vi "Blocking Performance Test Managment.vi"() -> ()   [LabVIEW 2013]
doc: "This VI will run the blobking performance tests at all required blocking frequency. See the below pseudo code for a description of its operation.\n\n1. Two test signals are fed to the EUT (equipment under test) input port: \na. Wanted signal: \ni. Modulated carrier, packets transmitted at the mid operating frequency = 2426 \nMHz, with 37-octets PRBS9 (pseudo random bit sequence 9) payload. Signal \nlevel of the wanted signal at the EUT input port shall be as defined below. \nb. Blocking signal: \ni. Sinusoidal, un-modulated carrier transmitted at a blocker frequency of fblocker \n= 30MHz. Signal level of the blocker signal at the EUT input port shall be as \ndefined in Table 1. \n2. If the PER (packet error rate) exceeds the minimum requirement, the frequency is recorded as \nfbf_1. \n3. Repeat steps for 1) and 2) for 30MHz = fblocker = 12.75GHz with the measurement \nfrequency resolution defined in Table 1. \n4. fblocker n+1 = fblocker_n + measurement frequency resolution (n=0,1,2…). \n5. The PER measurement is repeated for all recorded frequencies in 2) but with -50dBm blocker \nlevel at the EUT input ports. If the PER exceeds the minimum requirement, the frequency is \nrecorded as fbf_2. \nInterference signal frequency | Wanted signal level at EUT input port | Blocking signal level at EUT input port | Measurement frequency resolution \n30 – 2000 MHz | -67dBm | -30dBm | 10 MHz \n2003 – 2399 MHz | -67dBm | -35dBm | 3 MHz \n2484 – 2997 MHz | -67dBm | -35dBm | 3 MHz \n3000 MHz – 12.75 GHz | -67dBm | -30dBm | 25 MHz"
uses:
  Sub VIs/Master Test Parameters.ctl
  Sub VIs/Test Results Display Cluster.ctl
  Sub VIs/Pass Weighting.ctl
  Sub VIs/Test Managment Application Queue Control Cluster.ctl
  Sub VIs/Test Managment Application Queue Control.ctl
  Sub VIs/Results FGV Command.ctl
  Sub VIs/UUT Control Command.ctl
  Sub VIs/Test Parameters.ctl
  Sub VIs/Globals/Test Criteria Global.vi
panel:
  in  "Speed Throttle":bool
  out "Packets Sent":dbl format="%#.0f%%"
  in  "Result Emulation":T1=enum."Random"
  out "PER Pass Rate":dbl min=0.0 max=100.0 format="%#_g%%"
  out "Testing In Progress":bool
  out "State":string caption="Current Application State"
  out "Test Result":bool
  out "fbf_2 Pass Criteria":i32
  out "fbf_1 Pass Criteria":i32
  out "fbf_2":i32 caption="fbf_2 Results"
  out "fbf_1":i32 caption="fbf_1 Results"
  out "Array of Results":T2[](array[typedef]) {"Percentage Error Rates" format="%.1f%%"; "Test Frequency" format="%.0f MHz"}
  out "Freq. Under Test":u32 caption="Current frequency Under Test" format="%.0fMHz"
  out "Array of tests":T3[](array[typedef]) {"Measurement Res." format="%.0f MHz"; "Blocking Signal" format="%#_gdBm"; "Wanted Signal" format="%#_gdBm"; "Upper Frequency" format="%.0f MHz"; "Lower Frequency" format="%.0f MHz"}
  # "Blocking Performance Automated Test"
  # "Test Freq."
  # "Rcved Packets"
  # "Result"
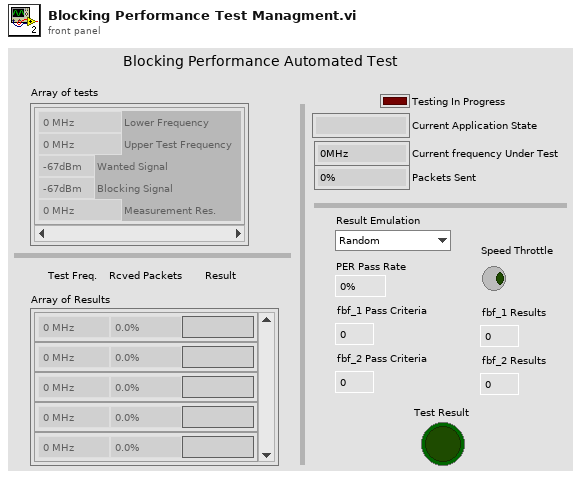
[diagram p1: front panel]
types:
  T1 = typedef "Pass Weighting.ctl" = enum16{"Always Pass", "Always Fail", "Always 30%", "Always 31%", "Random"}
  T2 = typedef "Test Results Display Cluster.ctl" = cluster{"Test Frequency":u32, "Percentage Error Rates":dbl, "Results":string}
  T3 = typedef "Master Test Parameters.ctl" = cluster{"Lower Frequency":u32, "Upper Frequency":u32, "Wanted Signal":dbl, "Blocking Signal":dbl, "Measurement Res.":u32}
  T4 = typedef "Test Managment Application Queue Control Cluster.ctl" = cluster{"State":T5, "Data":string}
  T5 = typedef "Test Managment Application Queue Control.ctl" = enum16{"Initialise", "Read Test Parameters", "Check for Correct UUT", "Round 1", "Set Blocking Signal Level", "Round 2", "Return Results", "Store Results", "End"}
  T6 = typedef "Results FGV Command.ctl" = enum16{"Add Result", "Return All", "Return fbf_1", "Return fbf_2", "Replace", "Clear All"}
  T7 = typedef "UUT Control Command.ctl" = enum16{"Initialise packet count", "Read Packet Count", "Return Temperature", "Return Operating Voltage"}
  T8 = typedef "Test Parameters.ctl" = cluster{"Interference sig. freq.":u32, "Wanted Signal":dbl, "Blocking Signal":dbl, "Measurement res.":u32}
  T9 = typedef "Test Results Cluster.ctl" = cluster{"Test Frequency":u32, "Received Packets":u32, "Results":string, "Test Paramaters":T8}
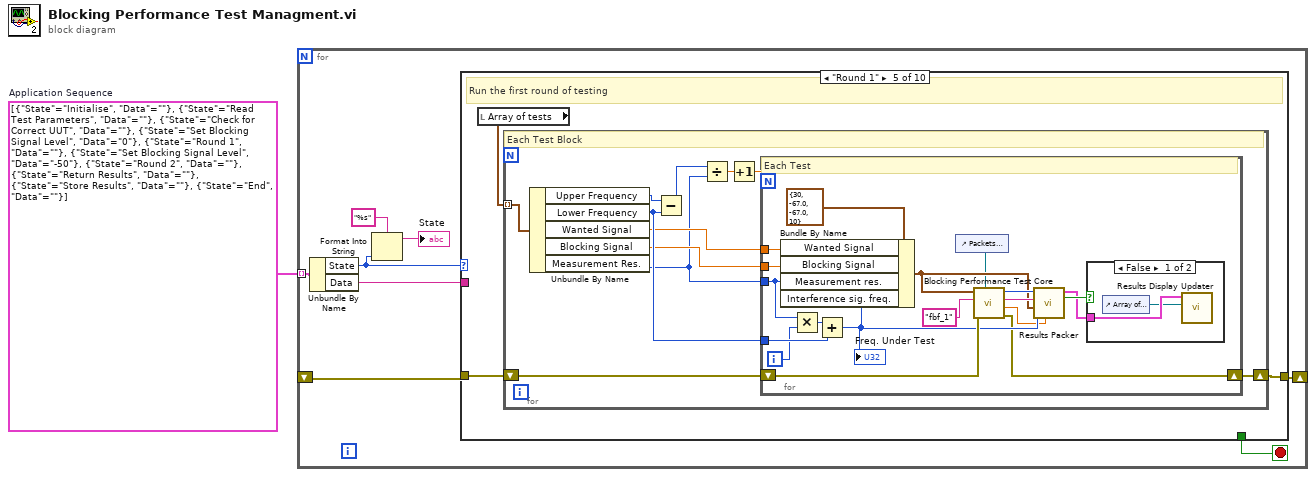
[diagram p0: block diagram]
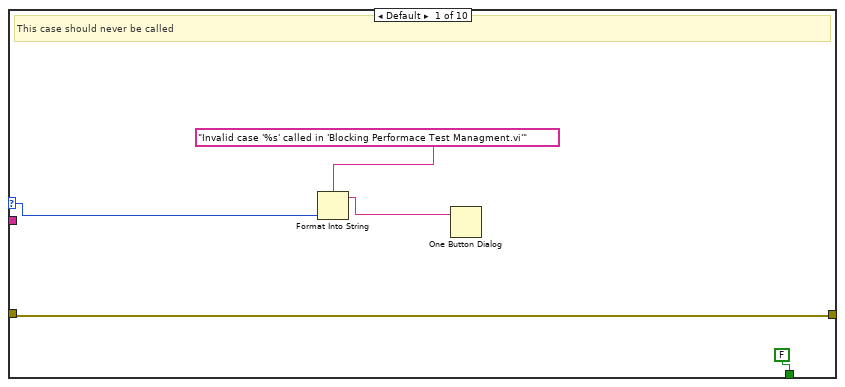
[diagram p2: hidden frame]
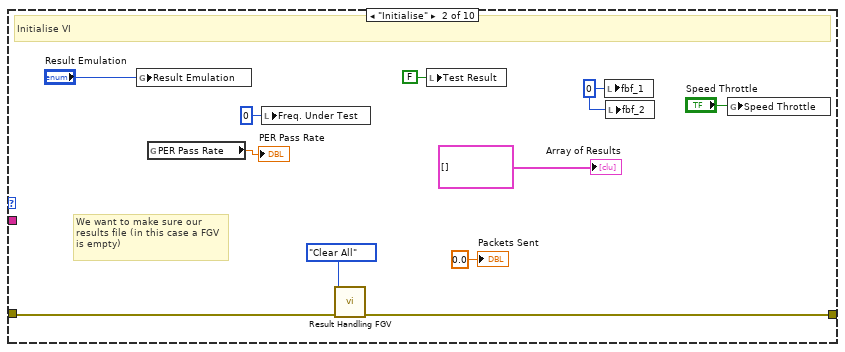
[diagram p3: hidden frame]
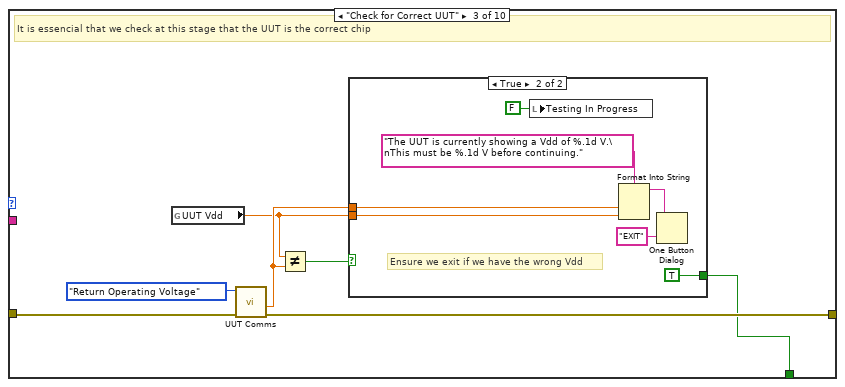
[diagram p4: hidden frame]
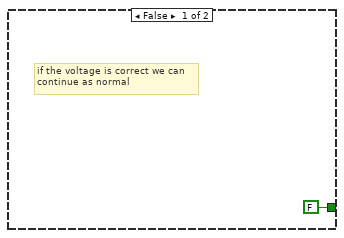
[diagram p5: hidden frame]
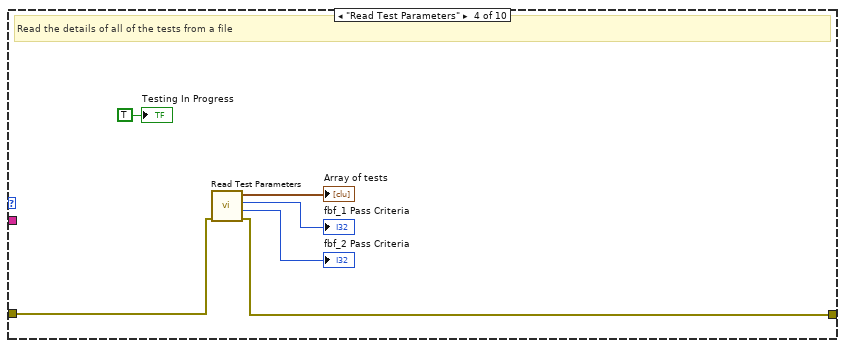
[diagram p6: hidden frame]
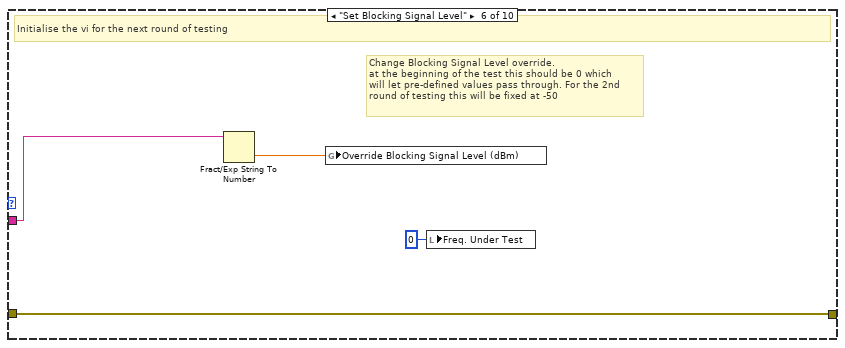
[diagram p8: hidden frame]
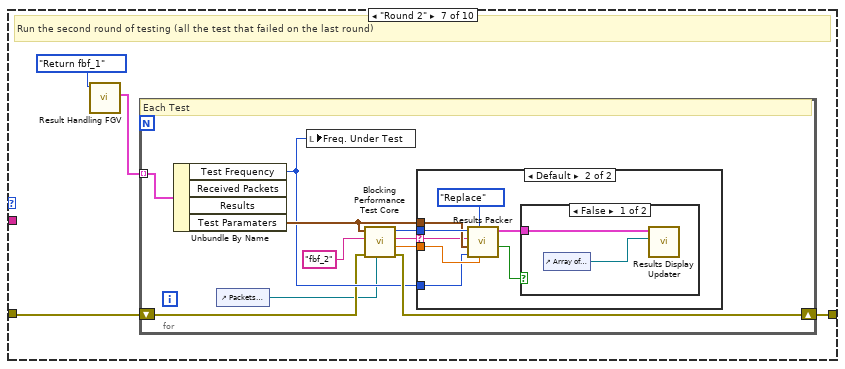
[diagram p9: hidden frame]
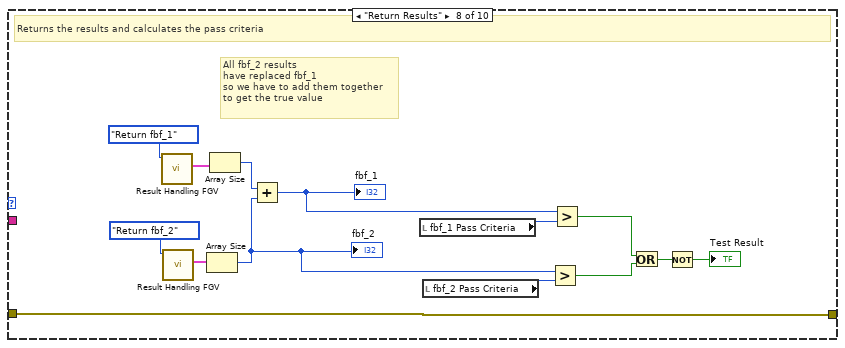
[diagram p12: hidden frame]
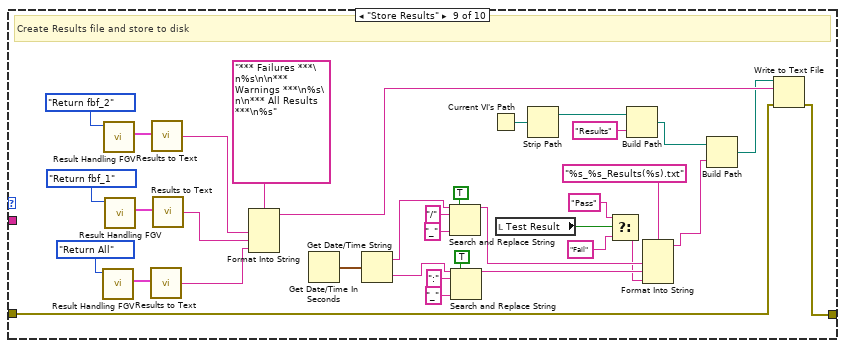
[diagram p13: hidden frame]
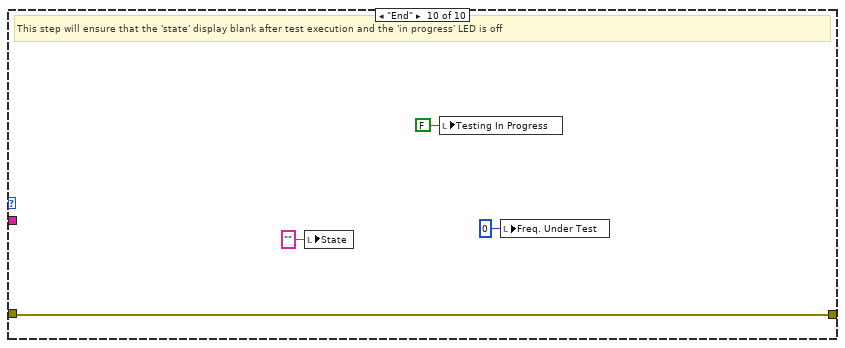
[diagram p14: hidden frame]
diagram:
  w1 = T4[] [{"State"=enum."Initialise", "Data"=""}, {"State"=enum."Read Test Parameters", "Data"=""}, {"State"=enum."Check for Correct UUT", "Data"=""}, {"State"=enum."Set Blocking Signal Level", "Data"="0"}, {"State"=enum."Round 1", "Data"=""}, {"State"=enum."Set Blocking Signal Level", "Data"="-50"}, {"State"=enum."Round 2", "Data"=""}, {"State"=enum."Return Results", "Data"=""}, {"State"=enum."Store Results", "Data"=""}, {"State"=enum."End", "Data"=""}]  # Application Sequence
  n1 = for {
    shift-right: [w9] -> _
    shift-left: _ -> [w8]
    tunnel: w1 -> [w6] mode=indexing
    stop <- w7 stop-if-true
    n2 = Unbundle By Name(w6) -> ("State"=w3:T5, "Data"=w4:string)
    n3 = Format Into String(format string="%s", w3) -> (resulting string=→"State":string)  [unwired: 2 in, 1 out]
    n4 = case shown="\"Round 1\"" w3 {
      selector: w3 -> [w11 _ _ _ _ _ _ _ _ _]
      tunnel: [w14 w23 w30 w44 w48 w83 w88 w111 w126 w161] -> w9
      tunnel: w8 -> [w14 w24 w31 w45 w47 w83 w87 w111 w127 w161]
      tunnel: [FALSE _ w28 _ _ _ _ _ _ _] -> w7
      tunnel: w4 -> [_ _ _ _ _ w82 _ _ _ _]
      frame Default {
        # "This case should never be called"
        n5 = Format Into String(format string="Invalid case '%s' called in 'Blocking Performace Test Managment.vi'" ("message"), w11) -> (resulting string=w12:string)  [unwired: 2 in, 1 out]
        n6 = One Button Dialog(message=w12) -> ()  [unwired: 1 in, 1 out]
      }
      frame "Initialise" {
        w21 = 0 ("fbf_1")
        # "We want to make sure our\nresults file (in this case a FGV\nis empty)"
        # "Initialise VI"
        n7 = global write "Test Criteria Global.vi" "Result Emulation"("Result Emulation") -> ()
        n8 = global read "Test Criteria Global.vi" "PER Pass Rate"() -> (→"PER Pass Rate":dbl)
        n9 = local write "Freq. Under Test"(u32 0 ("Freq. Under Test")) -> ()
        n10 = call "Result Handling FGV.vi"("error in"=w24, "Command"=Results_FGV_Command."Clear All") -> ("error out"=w23:errorcluster)  [unwired: 8 in, 1 out]
        n11 = local write "Test Result"(FALSE ("Test Result")) -> ()
        n12 = local write "fbf_1"(w21) -> ()
        n13 = local write "fbf_2"(w21) -> ()
        n14 = global write "Test Criteria Global.vi" "Speed Throttle"("Speed Throttle") -> ()
        "Packets Sent" <- 0.0 ("Packets Sent")
        "Array of Results" <- T2[] [] ("Results (Disp.)")
      }
      frame "Check for Correct UUT" {
        # "It is essencial that we check at this stage that the UUT is the correct chip"
        n15 = global read "Test Criteria Global.vi" "UUT Vdd"() -> (w26:dbl)
        n16 = call "UUT Comms.vi"("error in"=w31, "Command"=UUT_Control_Command."Return Operating Voltage") -> ("error out"=w30:errorcluster, "Vdd"=w27:dbl)  [unwired: 6 in, 2 out]
        n17 = Not Equal?(x=w26, y=w27) -> (x != y?=w29:bool)
        n18 = case shown="True" w29 {
          tunnel: [FALSE TRUE] -> w28
          tunnel: w27 -> [_ w36]
          tunnel: w26 -> [_ w35]
          frame False {
            # "if the voltage is correct we can\ncontinue as normal"
          }
          frame True {
            # "Ensure we exit if we have the wrong Vdd"
            n19 = local write "Testing In Progress"(FALSE ("Testing In Progress")) -> ()
            n20 = Format Into String(format string="The UUT is currently showing a Vdd of %.1d V.\nThis must be %.1d V before continuing.", w36, w35) -> (resulting string=w37:string)  [unwired: 2 in, 1 out]
            n21 = One Button Dialog(message=w37, button name ("OK")="EXIT") -> ()  [unwired: 1 out]
          }
        }
      }
      frame "Read Test Parameters" {
        # "Read the details of all of the tests from a file"
        n22 = call "Read Test Parameters.vi"("error in"=w45) -> ("error out"=w44:errorcluster, "fbf_2 Pass Criteria"=→"fbf_2 Pass Criteria":i32, "fbf_1 Pass Criteria"=→"fbf_1 Pass Criteria":i32, "Array of tests"=→"Array of tests":T3[])  [unwired: 7 in]
        "Testing In Progress" <- TRUE ("Testing In Progress")
      }
      frame "Round 1" {
        # "Run the first round of testing"
        n23 = local read "Array of tests"() -> (w49:T3[])
        n24 = for {
          tunnel: w49 -> [w60] mode=indexing
          shift-right: [w55] -> w48
          shift-left: w47 -> [w54]
          # "Each Test Block"
          n25 = Unbundle By Name(w60) -> ("Upper Frequency"=w59:u32, "Lower Frequency"=w58:u32, "Wanted Signal"=w57:dbl, "Blocking Signal"=w56:dbl, "Measurement Res."=w52:u32)
          n26 = Subtract(x=w59, y=w58) -> (x-y=w53:u32)
          n27 = Divide(x=w53, y=w52) -> (x/y=w51:dbl)
          n28 = Increment(x=w51) -> (x+1=w50:dbl)
          n29 = for {
            N: w50 -> [_]
            tunnel: w58 -> [w78]
            tunnel: w57 -> [w77]
            tunnel: w56 -> [w76]
            tunnel: w52 -> [w74]
            shift-right: [w65] -> w55
            shift-left: w54 -> [w75]
            i -> [w73]
            # "Each Test"
            n30 = Multiply(x=w74, y=w73) -> (x*y=w72:u32)
            n31 = Add(x=w72, y=w78) -> (x+y=w68:u32)
            "Freq. Under Test" <- w68
            n32 = Bundle By Name(cluster=T8 {"Interference sig. freq."=30, "Wanted Signal"=-67.0, "Blocking Signal"=-67.0, "Measurement res."=10} ("Test Paramaters"), "Wanted Signal"=w77, "Blocking Signal"=w76, "Measurement res."=w74, "Interference sig. freq."=w68) -> (w67:T8)
            n33 = control-ref of="Packets Sent"() -> (w62:refnum<vi>)
            n34 = call "Blocking Performance Test Core.vi"("Packets Sent"=w62, "error in"=w75, "test run"="fbf_1", "Test Paramaters"=w67) -> ("error out"=w65:errorcluster, "PER"=w66:dbl, "Results"=w71:string, "received Packets"=w70:u32)  [unwired: 4 in]
            n35 = call "Results Packer.vi"("PER"=w66, "Test Frequency"=w68, "Test Paramaters"=w67, "Results"=w71, "received Packets"=w70) -> ("Pass"=w64:bool, "Test Result Display Cluster"=w61:T2)  [unwired: 4 in, 1 out]
            n36 = case shown="False" w64 {
              tunnel: w61 -> [w80 _]
              frame False {
                n37 = control-ref of="Array of Results"() -> (w79:refnum<vi>)
                n38 = call "Results Display Updater.vi"("Array of Results Reference"=w79, "New Results"=w80) -> ()  [unwired: 10 in]
              }
              frame True {
              }
            }
          }
        }
      }
      frame "Set Blocking Signal Level" {
        # "Change Blocking Signal Level override.\nat the beginning of the test this should be 0 which\nwill let pre-defined values pass through. For the 2nd\nround of testing this will be fixed at -50"
        # "Initialise the vi for the next round of testing"
        n39 = Fract/Exp String To Number(string=w82) -> (number=w81:dbl)  [unwired: 3 in, 1 out]
        n40 = global write "Test Criteria Global.vi" "Override Blocking Signal Level (dBm)"(w81) -> ()
        n41 = local write "Freq. Under Test"(u32 0 ("Freq. Under Test")) -> ()
      }
      frame "Round 2" {
        # "Run the second round of testing (all the test that failed on the last round)"
        n42 = call "Result Handling FGV.vi"("Command"=Results_FGV_Command."Return fbf_1") -> ("Result Array"=w85:T9[])  [unwired: 9 in, 1 out]
        n43 = for {
          shift-right: [w96] -> w88
          shift-left: w87 -> [w90]
          tunnel: w85 -> [w95] mode=indexing
          # "Each Test"
          n44 = Unbundle By Name(w95) -> ("Test Frequency"=w92:u32, "Test Paramaters"=w94:T8)  [unwired: 2 out]
          n45 = control-ref of="Packets Sent"() -> (w89:refnum<vi>)
          n46 = local write "Freq. Under Test"(w92) -> ()
          n47 = call "Blocking Performance Test Core.vi"("Packets Sent"=w89, "error in"=w90, "test run"="fbf_2", "Test Paramaters"=w94) -> ("error out"=w96:errorcluster, "PER"=w97:dbl, "Results"=w91:string, "received Packets"=w98:u32)  [unwired: 4 in]
          n48 = case shown="Default" w91 {
            selector: w91 -> [_ w101]
            tunnel: w98 -> [_ w106]
            tunnel: w97 -> [_ w105]
            tunnel: w94 -> [_ w104]
            tunnel: w92 -> [_ w103]
            frame "Pass" {
              # "If the test now\npasses we leave\nthe results alone"
            }
            frame Default {
              n49 = call "Results Packer.vi"("PER"=w105, "Command (Add)"=Results_FGV_Command."Replace" ("Command"), "Test Frequency"=w103, "Test Paramaters"=w104, "Results"=w101, "received Packets"=w106) -> ("Pass"=w100:bool, "Test Result Display Cluster"=w99:T2)  [unwired: 3 in, 1 out]
              n50 = case shown="False" w100 {
                tunnel: w99 -> [w108 _]
                frame False {
                  n51 = control-ref of="Array of Results"() -> (w107:refnum<vi>)
                  n52 = call "Results Display Updater.vi"("Array of Results Reference"=w107, "New Results"=w108) -> ()  [unwired: 10 in]
                }
                frame True {
                  # "Do not display the results\nif they are true, IE only show\ntest failures"
                }
              }
            }
          }
        }
      }
      frame "Return Results" {
        # "All fbf_2 results\nhave replaced fbf_1\nso we have to add them together\nto get the true value"
        # "Returns the results and calculates the pass criteria"
        n53 = call "Result Handling FGV.vi"("Command"=Results_FGV_Command."Return fbf_1") -> ("Result Array"=w120:T9[])  [unwired: 9 in, 1 out]
        n54 = call "Result Handling FGV.vi"("Command"=Results_FGV_Command."Return fbf_2") -> ("Result Array"=w119:T9[])  [unwired: 9 in, 1 out]
        n55 = Array Size(array=w119) -> (size(s)=w116:i32)
        "fbf_2" <- w116
        n56 = Array Size(array=w120) -> (size(s)=w118:i32)
        n57 = Add(x=w118, y=w116) -> (x+y=w117:i32)
        "fbf_1" <- w117
        n58 = local read "fbf_1 Pass Criteria"() -> (w110:i32)
        n59 = local read "fbf_2 Pass Criteria"() -> (w109:i32)
        n60 = Greater?(x=w116, y=w109) -> (0:w114:bool)
        n61 = Greater?(x=w117, y=w110) -> (0:w115:bool)
        n62 = Or(x=w115, y=w114) -> (x .or. y?=w113:bool)
        n63 = Not(x=w113) -> (.not. x?=→"Test Result":bool)
      }
      frame "Store Results" {
        # "Create Results file and store to disk"
        n64 = call "Result Handling FGV.vi"("Command"=Results_FGV_Command."Return All") -> ("Result Array"=w151:T9[])  [unwired: 9 in, 1 out]
        n65 = call "Result Handling FGV.vi"("Command"=Results_FGV_Command."Return fbf_2") -> ("Result Array"=w156:T9[])  [unwired: 9 in, 1 out]
        n66 = call "Result Handling FGV.vi"("Command"=Results_FGV_Command."Return fbf_1") -> ("Result Array"=w154:T9[])  [unwired: 9 in, 1 out]
        n67 = call "Results to Text.vi"("Result Array"=w151) -> ("String"=w148:string)
        n68 = call "Results to Text.vi"("Result Array"=w156) -> ("String"=w150:string)
        n69 = call "Results to Text.vi"("Result Array"=w154) -> ("String"=w149:string)
        n70 = Format Into String(format string="*** Failures ***\n%s\n\n*** Warnings ***\n%s\n\n*** All Results ***\n%s", w150, w149, w148) -> (resulting string=w145:string)  [unwired: 2 in, 1 out]
        n71 = Get Date/Time In Seconds() -> (seconds since 1Jan1904=w146:timestamp)
        n72 = Get Date/Time String(seconds (now)=w146) -> (date string=w137:string, time string=w141:string)  [unwired: 2 in]
        n73 = Search and Replace String(replace all?=TRUE ("replace all? (F)"), input string=w137, search string="/", replace string="_" ("replace string (\"\")")) -> (result string=w135:string)  [unwired: 4 in, 3 out]
        n74 = Search and Replace String(replace all?=TRUE ("replace all? (F)"), input string=w141, search string=":", replace string="_" ("replace string (\"\")")) -> (result string=w134:string)  [unwired: 4 in, 3 out]
        n75 = Current VI's Path() -> (path=w147:path)
        n76 = local read "Test Result"() -> (w131:bool)
        n77 = Strip Path(path=w147) -> (stripped path=w125:path)  [unwired: 1 out]
        n78 = Select(t="Pass", s=w131, f="Fail") -> (s? t:f=w130:string)
        n79 = Build Path(base path=w125, name or relative path="Results") -> (appended path=w124:path)
        n80 = Format Into String(format string="%s_%s_Results(%s).txt", w135, w134, w130) -> (resulting string=w129:string)  [unwired: 2 in, 1 out]
        n81 = Build Path(base path=w124, name or relative path=w129) -> (appended path=w128:path)
        n82 = Write to Text File(file (use dialog)=w128, text=w145, error in=w127) -> (error out=w126:errorcluster)  [unwired: 1 in, 2 out]
      }
      frame "End" {
        # "This step will ensure that the 'state' display blank after test execution and the 'in progress' LED is off"
        n83 = local write "State"("" ("State")) -> ()
        n84 = local write "Testing In Progress"(FALSE ("Testing In Progress")) -> ()
        n85 = local write "Freq. Under Test"(u32 0 ("Freq. Under Test")) -> ()
      }
    }
  }
